vi "get desired keys.vi"(8 "error in":errorcluster, 11 "My Awesome Control Modules configuration in":refnum<class "My Awesome Control Modules configuration.lvclass">) -> (0 "error out":errorcluster, 2 "desired keys":string[](array[string]), 3 "My Awesome Control Modules configuration out":refnum<class "My Awesome Control Modules configuration.lvclass">)   [LabVIEW 2013, in "My Awesome Control Modules configuration.lvclass"]
uses:
  My Awesome Control Modules configuration.lvclass
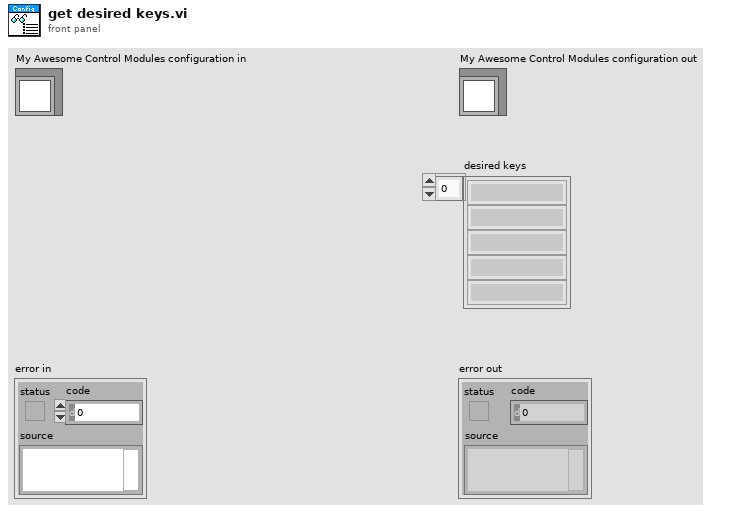
[diagram p1: front panel]
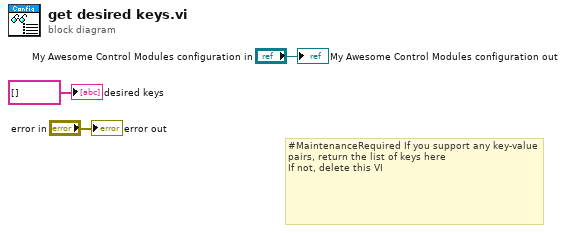
[diagram p0: block diagram]
diagram:
  # "#MaintenanceRequired If you support any key-value pairs, return the list of keys here\nIf not, delete this VI"
  "error out" <- "error in"
  "My Awesome Control Modules configuration out" <- "My Awesome Control Modules configuration in"
  "desired keys" <- string[] [] ("desired keys")
